vi "Kinect Standardize Cropped Image.vi"(9 "Height":i32=100, 10 "Width":i32=100, 11 "Image":T1(plugin-control)) -> (2 "Image Dst Out":T1(plugin-control), 3 "Image Original Out":T1)   [LabVIEW 2011]
uses:
  <vilib>/vision/Image Controls.llb/IMAQ Image.ctl
  <vilib>/vision/NI_Vision_Development_Module.lvlib
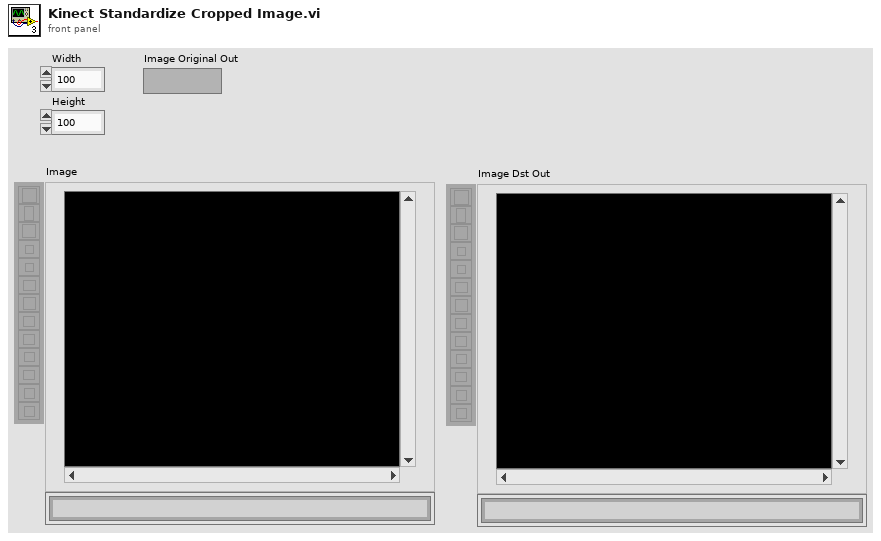
[diagram p1: front panel]
types:
  T1 = typedef "IMAQ Image.ctl" = refnum<image>
  T2 = typedef "Image Type" = u32
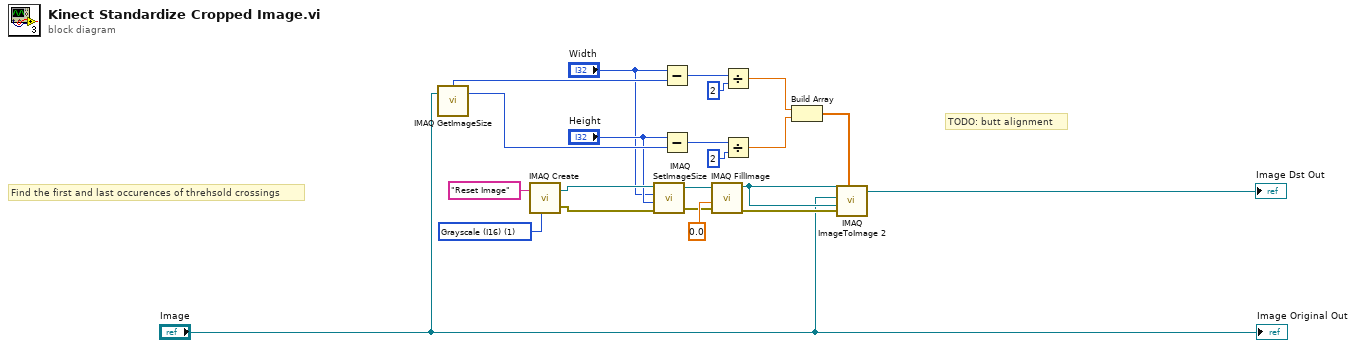
[diagram p0: block diagram]
diagram:
  w19 = T2 1 items=["Grayscale (U8)", "Grayscale (I16)", "Grayscale (SGL)", "Complex (CSG)", "RGB (U32)", "HSL (U32)", "RGB (U64)", "Grayscale (U16)"] ("Image Type")
  # "Find the first and last occurences of threhsold crossings"
  # "TODO: butt alignment"
  n1 = call "IMAQ GetImageSize"("Image"="Image") -> ("Y Resolution"=w12:i32, "X Resolution"=w13:i32)  [unwired: 3 in, 1 out]
  n2 = call "IMAQ Create"("Image Name"="Reset Image", "Image Type"=w19) -> ("New Image"=w10:T1, "error out"=w9:errorcluster)  [unwired: 3 in]
  n3 = call "IMAQ SetImageSize"("error in (no error)"=w9, "Y Resolution"="Height", "X Resolution"="Width", "Image"=w10) -> ("error out"=w6:errorcluster, "Image Out"=w8:T1)  [unwired: 1 in]
  n4 = Subtract(x="Width", y=w13) -> (x-y=w17:i32)
  n5 = Subtract(x="Height", y=w12) -> (x-y=w18:i32)
  n6 = call "IMAQ FillImage"("error in (no error)"=w6, "Pixel Value (U8, U16, I16, Float)"=sgl 0.0, "Image"=w8) -> ("error out"=w5:errorcluster, "Image Out"=w4:T1)  [unwired: 7 in]
  n7 = Divide(x=w17, y=2) -> (x/y=w16:dbl)
  n8 = Divide(x=w18, y=2) -> (x/y=w15:dbl)
  n9 = Build Array(w16, w15) -> (w14:dbl[])
  n10 = call "IMAQ ImageToImage 2"("Offset Left/Top"=w14, "error in (no error)"=w5, "Image Dst"=w4, "Image Src (Small)"="Image", "Image Src (Large)"=w4) -> ("Image Dst Out"=→"Image Dst Out":T1)  [unwired: 5 in, 1 out]
  "Image Original Out" <- "Image"
